vi "HSCAN.vi"(4 "count":i64, 6 "MATCH pattern":string, 7 "TYPE":string, 8 "error in (no error)":errorcluster, 9 "cursor":i64, 10 "key":string, 11 "Redis Client in":refnum<class "Redis Client.lvclass">) -> (0 "error out":errorcluster, 2 "RESP3 Value":variant, 3 "Redis Client out":refnum<class "Redis Client.lvclass">)   [LabVIEW 2019, in "Redis Client for LabVIEW.lvlib" / "Redis Client.lvclass"]
uses:
  Redis Client.lvclass
  lib/RESP3-for-LabVIEW/RESP3/subVIs/RESP3 Make String Base.vi
  lib/RESP3-for-LabVIEW/RESP3/types/RESP3 data type attribute.vi
  lib/RESP3-for-LabVIEW/RESP3/RESP3.lvlib
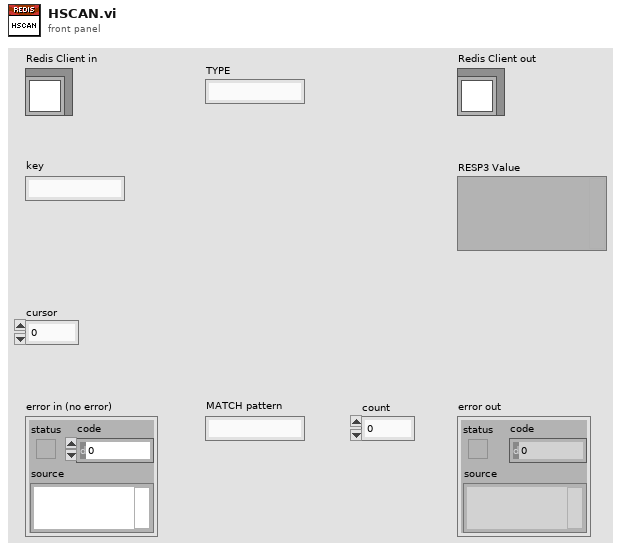
[diagram p1: front panel]
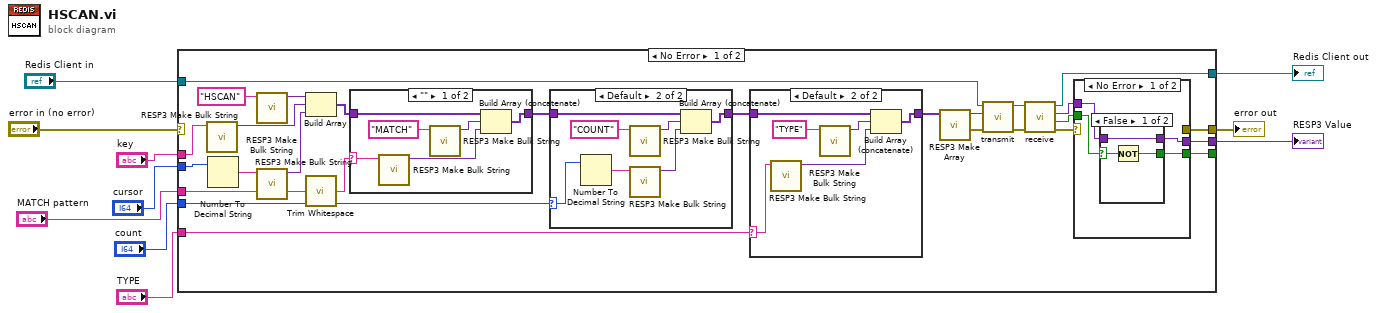
[diagram p0: block diagram]
diagram:
  n1 = case shown="No Error" "error in (no error)" {
    selector: "error in (no error)" -> [_ w69]
    tunnel: [w24 w69] -> w9
    tunnel: "Redis Client in" -> [w37 w68]
    tunnel: [w35 w68] -> w7
    tunnel: "key" -> [w32 _]
    tunnel: "cursor" -> [w31 _]
    tunnel: [w23 _] -> _
    tunnel: [w20 _] -> w4
    tunnel: "MATCH pattern" -> [w18 _]
    tunnel: "count" -> [w15 _]
    tunnel: "TYPE" -> [w11 _]
    frame No Error {
      n2 = call "RESP3 Make Bulk String.vi"("String"=w32) -> ("RESP3 Value out"=w29:variant)  [unwired: 9 in, 1 out]
      n3 = Number To Decimal String(number=w31) -> (decimal integer string=w19:string)  [unwired: 1 in]
      n4 = call "RESP3 Make Bulk String.vi"("String"="HSCAN" ("string in")) -> ("RESP3 Value out"=w30:variant)  [unwired: 9 in, 1 out]
      n5 = call "RESP3 Make Bulk String.vi"("String"=w19) -> ("RESP3 Value out"=w28:variant)  [unwired: 9 in, 1 out]
      n6 = Build Array(w30, w29, w28) -> (w16:variant[])
      n7 = call <vilib>:"Trim Whitespace.vi"("string"=w18) -> ("trimmed string"=w17:string)  [unwired: 1 in]
      n8 = case shown="\"\"" w17 {
        selector: w17 -> [w57 _]
        tunnel: w16 -> [w56 w59]
        tunnel: [w53 w59] -> w14
        frame "" {
          n9 = call "RESP3 Make Bulk String.vi"("String"=w57) -> ("RESP3 Value out"=w54:variant)  [unwired: 9 in, 1 out]
          n10 = call "RESP3 Make Bulk String.vi"("String"="MATCH") -> ("RESP3 Value out"=w55:variant)  [unwired: 9 in, 1 out]
          n11 = Build Array (concatenate)(w56, w55, w54) -> (w53:variant[])
        }
        frame Default {
        }
      }
      n12 = case shown="Default" w15 {
        selector: w15 -> [_ w51]
        tunnel: [w45 w48] -> w13
        tunnel: w14 -> [w45 w50]
        frame ..0 {
        }
        frame Default {
          n13 = Number To Decimal String(number=w51) -> (decimal integer string=w52:string)  [unwired: 1 in]
          n14 = call "RESP3 Make Bulk String.vi"("String"="COUNT") -> ("RESP3 Value out"=w47:variant)  [unwired: 9 in, 1 out]
          n15 = call "RESP3 Make Bulk String.vi"("String"=w52) -> ("RESP3 Value out"=w49:variant)  [unwired: 9 in, 1 out]
          n16 = Build Array (concatenate)(w50, w47, w49) -> (w48:variant[])
        }
      }
      n17 = case shown="Default" w11 {
        selector: w11 -> [_ w39]
        tunnel: [w38 w42] -> w12
        tunnel: w13 -> [w38 w44]
        frame "" {
        }
        frame Default {
          n18 = call "RESP3 Make Bulk String.vi"("String"=w39) -> ("RESP3 Value out"=w43:variant)  [unwired: 9 in, 1 out]
          n19 = call "RESP3 Make Bulk String.vi"("String"="TYPE") -> ("RESP3 Value out"=w41:variant)  [unwired: 9 in, 1 out]
          n20 = Build Array (concatenate)(w44, w41, w43) -> (w42:variant[])
        }
      }
      n21 = call "RESP3 Make Array.vi"("RESP3 Values in"=w12) -> ("error out"=w26:errorcluster, "RESP3 Value out"=w27:variant)  [unwired: 9 in]
      n22 = call-dynamic "transmit.vi"("error in (no error)"=w26, "RESP3 Value"=w27, "Redis Client in"=w37) -> ("error out"=w34:errorcluster, "Redis Client out"=w36:refnum<class "Redis Client.lvclass">)  [unwired: 7 in]
      n23 = call-dynamic "receive.vi"("error in (no error)"=w34, "Redis Client in"=w36) -> ("error out"=w22:errorcluster, "timed out?"=w21:bool, "RESP3 Value"=w25:variant, "Redis Client out"=w35:refnum<class "Redis Client.lvclass">)  [unwired: 6 in]
      n24 = case shown="No Error" w22 {
        selector: w22 -> [_ w67]
        tunnel: w25 -> [w63 _]
        tunnel: [_ w67] -> w24
        tunnel: [w62 _] -> w23
        tunnel: w21 -> [w61 _]
        tunnel: [w60 _] -> w20
        frame No Error {
          n25 = case shown="False" w61 {
            selector: w61 -> [w64 _]
            tunnel: w63 -> [w65 _]
            tunnel: [w66 _] -> w62
            tunnel: [w65 _] -> w60
            frame False {
              n26 = Not(x=w64) -> (.not. x?=w66:bool)
            }
            frame True {
            }
          }
        }
        frame Error {
        }
      }
    }
    frame Error {
    }
  }
  "error out" <- w9
  "Redis Client out" <- w7
  "RESP3 Value" <- w4
